vi "Read TDMS.vi"() -> ()   [LabVIEW 2020]
panel:
  out "Waveform Graph":waveform(dbl)(graph)
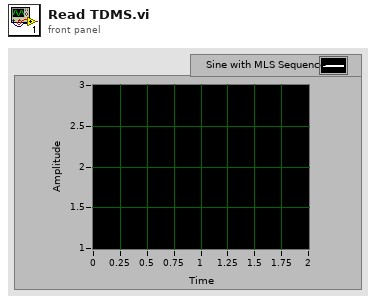
[diagram p1: front panel]
types:
  T1 = enum16{"open", "open or create", "create or replace", "create", "open (read-only)"}
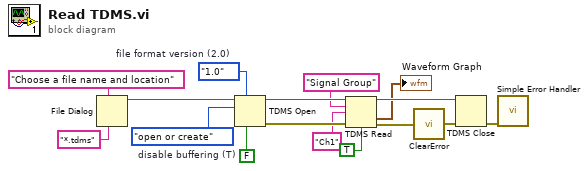
[diagram p0: block diagram]
diagram:
  w5 = enum16{"1.0", "2.0"}."1.0"  # file format version (2.0)
  w7 = FALSE  # disable buffering (T)
  n1 = File Dialog(6:"*.tdms" ("pattern (all files)"), 7:"Choose a file name and location" ("prompt")) -> (3:w12:path)  [unwired: 1 in, 7 out]
  n2 = TDMS Open(6:w7, 7:w5, 10:T1."open or create" ("operation"), 11:w12) -> (0:w8:errorcluster, 3:w9:refnum<k34>)  [unwired: 3 in]
  n3 = TDMS Read(0:w9, 5:"Signal Group" ("group name in"), 7:"Ch1" ("group name in"), 11:w8, 13:TRUE ("return channels in file order? (F)")) -> (4:w15:refnum<k34>, 10:→"Waveform Graph":waveform(dbl), 15:w6:errorcluster)  [unwired: 3 in, 3 out]
  n4 = call <vilib>:"ClearError.vi"("error in (no error)"=w6) -> ("error out"=w4:errorcluster)
  n5 = TDMS Close(8:w4, 11:w15) -> (0:w16:errorcluster)  [unwired: 1 out]
  n6 = call <vilib>:"Simple Error Handler.vi"("error in (no error)"=w16) -> ()  [unwired: 1 in, 8 out]
